vi "Keithley 2200 Series Monitor Output.vi"() -> ()   [LabVIEW 2024]
doc: "DESCRIPTION:\n\nThis VI configures the power supply to generate a DC voltage output.\nIt also displays the Output Voltage,Current ,Power,DVM and Resistance as per the selected parameter. \n\nINSTRUCTIONS:\n1. Enter the resource name.\n2. Enter voltage or current value to set the voltage or current value of the power supply .\n3. Set On/Off switch to Enable if you want the generated voltage to appear at the instrument's output. \n4. Select Local/Remote mode operation.If local command is select ,this will set the instrument in local mode.\n5.Select the parameter from the control,to read the responce from the instrument.\n6.Run the VI.\n\nNOTES:\nNotice the order of the power supply component VIs in the block diagram. The first VI in a sequence is the power supply Initialize.vi, which provides a VISA session to the instrument driver. The last VI in a sequence must be the power supply Close.vi which closes the Visa session."
uses:
  Keithley 2200 Series.lvlib
  Keithley DMM6500/Keithley DMM6500 DAQ6500 Series.lvlib
panel:
  in  "Function(0:Voltage)":u16(ring) items=["Voltage", "Current"]
  in  "Unit(V)":u16(ring) items=["V", "mV", "kV", "A", "mA"]
  in  "Measurement Function(0:Voltage)":u16(ring) items=["Voltage", "Current", "Power", "Digital Volt Meter", "Resistance"]
  in  "Control Mode(1:Remote)":u16(ring)=1 items=["Local", "Remote"]
  in  "Manual Range(0.00)":dbl format="%.2f"
  in  "Enable Output (T: Enable)":bool=TRUE
  out "Measurement":string
  in  "VISA resource name":refnum<visa-resource-name>
  # "(c) Copyright 2012 Keithley Instruments Inc  ALL RIGHTS RESERVED."
  # "Configure Instrument"
  # "Read Measurement"
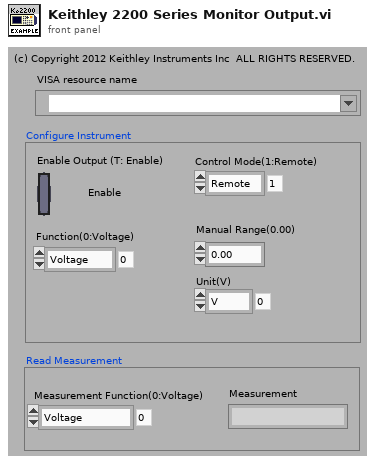
[diagram p1: front panel]
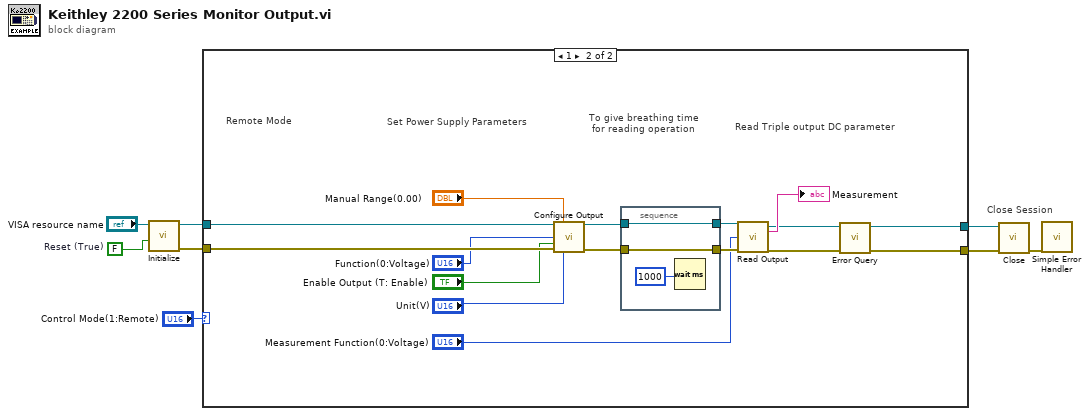
[diagram p0: block diagram]
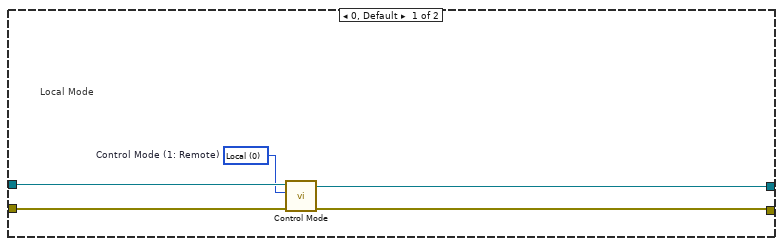
[diagram p2: hidden frame]
diagram:
  w1 = FALSE items=["OFF", "ON", "OFF", "ON"]  # Reset (True)
  # "Close Session"
  n1 = call "Initialize.vi"("Reset (True)"=w1, "VISA resource name"="VISA resource name") -> ("error out"=w2:errorcluster, "VISA resource name out"=w3:refnum<visa-resource-name>)  [unwired: 4 in, 4 out]
  n2 = case shown="1" "Control Mode(1:Remote)" {
    tunnel: [w10 w21] -> w4
    tunnel: w3 -> [w13 w25]
    tunnel: w2 -> [w12 w24]
    tunnel: [w9 w22] -> w6
    frame 0, Default {
      w11 = u16 0 items=["Local", "Remote", "Remote Lock"]  # Control Mode (1: Remote)
      # "Local Mode"
      n3 = call "Control Mode.vi"("error in (no error)"=w12, "Control Mode (1: Remote)"=w11, "VISA resource name"=w13) -> ("error out"=w10:errorcluster, "VISA resource name out"=w9:refnum<visa-resource-name>)  [unwired: 7 out]
    }
    frame 1 {
      # "Read Triple output DC parameter"
      # "To give breathing time\n for reading operation"
      # "Set Power Supply Parameters"
      # "Remote Mode"
      n4 = call "Configure Output.vi"("VISA resource name"=w25, "Manual Range(0.00)"="Manual Range(0.00)", "Function(0:Voltage)"="Function(0:Voltage)", "Enable Output (T: Enable)"="Enable Output (T: Enable)", "error in (no error)"=w24, "Unit(V)"="Unit(V)") -> ("VISA resource name out"=w29:refnum<visa-resource-name>, "error out"=w27:errorcluster)  [unwired: 8 out]
      n5 = stacked-sequence {
        tunnel: w29 -> [w31]
        tunnel: [w31] -> w28
        tunnel: w27 -> [w30]
        tunnel: [w30] -> w26
        frame #0 {
          n6 = Wait (ms)(milliseconds to wait=u32 1000 ("millisecond multiple")) -> ()  [unwired: 1 out]
        }
      }
      n7 = call "Read Output.vi"("VISA resource name"=w28, "Measurement Function (0:Voltage)"="Measurement Function(0:Voltage)", "error in (no error)"=w26) -> ("VISA resource name out"=w17:refnum<visa-resource-name>, "Measurement"=→"Measurement":string, "error out"=w16:errorcluster)  [unwired: 10 out]
      n8 = call "Error Query.vi"("error in (no error)"=w16, "VISA resource name"=w17) -> ("error out"=w21:errorcluster, "VISA resource name out"=w22:refnum<visa-resource-name>)  [unwired: 8 out]
    }
  }
  n9 = call "Close.vi"("error in (no error)"=w4, "VISA resource name"=w6) -> ("error out"=w5:errorcluster)  [unwired: 9 out]
  n10 = call <vilib>:"Simple Error Handler.vi"("error in (no error)"=w5) -> ()  [unwired: 1 in, 8 out]
